vi "19.1-MovingAverage-Window.vi"() -> ()   [LabVIEW 2020]
doc: "This example demonstrates the importance of using windows when performing spectral analysis on signals which contain multiple frequencies.\n\nThe effect of different types of window functions is shown in the frequency domain. With no window function used, Sine Wave 2 buries the low amplitude Sine Wave 1. Using the Hanning Window (Window 2), the smaller signal can be detected."
uses:
  <vilib>/Analysis/0measdsp.llb/Scaled Time Domain Window (DBL).vi
  <vilib>/Analysis/NI_AALPro.lvlib
panel:
  out "H[k]":dbl[][](graph)
  out "H[k]-dB":dbl[][](graph)
  out "h[n]":dbl[][](graph)
  in  "window 1":u32(ring)=5 items=["Rectangle"=0, "Hanning"=1, "Hamming"=2, "Blackman-Harris"=3, "Exact Blackman"=4, "Blackman"=5, "Flat Top"=6, "4 Term B-Harris "=7, "7 Term B-Harris"=8, "Low Sidelobe"=9, "Blackman Nuttall"=11, "Triangle"=30, "Bartlett-Hanning"=31, "Bohman"=32, "Parzen"=33, "Welch"=34, "Kaiser"=60, "Dolph-Chebyshev"=61, "Gaussian"=62]
  in  "window 2":u32(ring)=62 items=["Rectangle"=0, "Hanning"=1, "Hamming"=2, "Blackman-Harris"=3, "Exact Blackman"=4, "Blackman"=5, "Flat Top"=6, "4 Term B-Harris "=7, "7 Term B-Harris"=8, "Low Sidelobe"=9, "Blackman Nuttall"=11, "Triangle"=30, "Bartlett-Hanning"=31, "Bohman"=32, "Parzen"=33, "Welch"=34, "Kaiser"=60, "Dolph-Chebyshev"=61, "Gaussian"=62]
  in  "Stop":bool
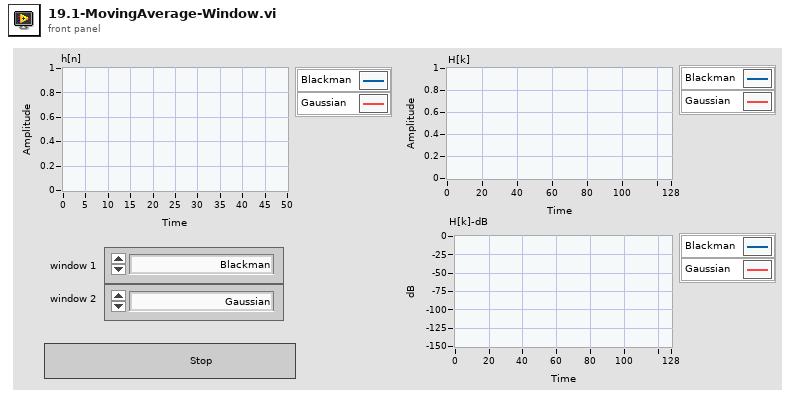
[diagram p1: front panel]
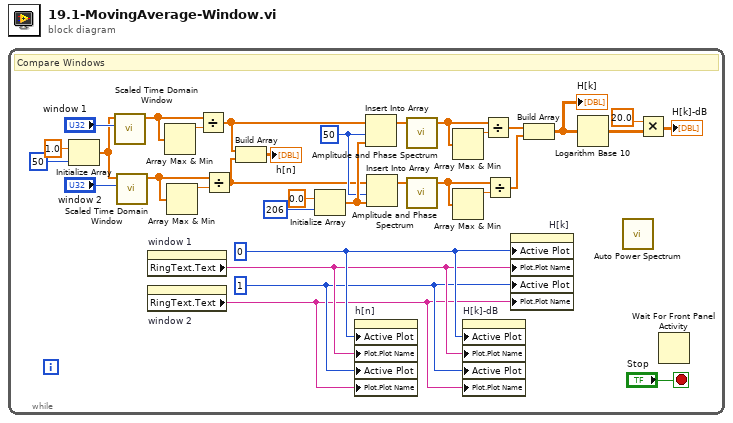
[diagram p0: block diagram]
diagram:
  n1 = while {
    stop <- "Stop" stop-if-true
    w17 = 50 ("index")
    w4 = u32 0
    w2 = u32 1 ("Active Plot")
    # "Compare Windows"
    n2 = Initialize Array(1.0 ("element"), 50 ("dimension size")) -> (w28:dbl[])
    n3 = call-poly <vilib>:"Scaled Time Domain Window.vi"("window"="window 1", "X"=w28) -> ("Windowed X"=w25:dbl[])  [unwired: 7 in, 2 out]
    n4 = call-poly <vilib>:"Scaled Time Domain Window.vi"("window"="window 2", "X"=w28) -> ("Windowed X"=w23:dbl[])  [unwired: 7 in, 2 out]
    n5 = property on="window 1" class="Ring (strict)"() -> ("RingText.Text"=w3:string)  [unwired: 2 in, 2 out]
    n6 = property on="window 2" class="Ring (strict)"() -> ("RingText.Text"=w1:string)  [unwired: 2 in, 2 out]
    n7 = Array Max & Min(array=w25) -> (max value=w26:dbl)  [unwired: 3 out]
    n8 = Array Max & Min(array=w23) -> (max value=w24:dbl)  [unwired: 3 out]
    n9 = Divide(x=w25, y=w26) -> (x/y=w16:dbl[])
    n10 = Divide(x=w23, y=w24) -> (x/y=w15:dbl[])
    n11 = Build Array(w16, w15) -> (→"h[n]":dbl[][])
    n12 = Initialize Array(0.0 ("element"), 206 ("dimension size")) -> (w18:dbl[])
    n13 = property on="h[n]" class="WFGraph (strict)"("Active Plot"=w4, "Plot.Plot Name"=w3, "Active Plot"=w2, "Plot.Plot Name"=w1) -> ()  [unwired: 2 in, 2 out]
    n14 = Insert Into Array(array=w16, index=w17, new element=w18) -> (w12:dbl[])
    n15 = Insert Into Array(array=w15, index=w17, new element=w18) -> (w11:dbl[])
    n16 = call <vilib>:"Amplitude and Phase Spectrum.vi"("Signal (V)"=w12) -> ("Amp Spectrum Mag (Vrms)"=w8:dbl[])  [unwired: 2 in, 2 out]
    n17 = call <vilib>:"Amplitude and Phase Spectrum.vi"("Signal (V)"=w11) -> ("Amp Spectrum Mag (Vrms)"=w7:dbl[])  [unwired: 2 in, 2 out]
    n18 = Array Max & Min(array=w8) -> (max value=w13:dbl)  [unwired: 3 out]
    n19 = Array Max & Min(array=w7) -> (max value=w14:dbl)  [unwired: 3 out]
    n20 = property on="H[k]-dB" class="WFGraph (strict)"("Active Plot"=w4, "Plot.Plot Name"=w3, "Active Plot"=w2, "Plot.Plot Name"=w1) -> ()  [unwired: 2 in, 2 out]
    n21 = Divide(x=w8, y=w13) -> (x/y=w6:dbl[])
    n22 = Divide(x=w7, y=w14) -> (x/y=w5:dbl[])
    n23 = property on="H[k]" class="WFGraph (strict)"("Active Plot"=w4, "Plot.Plot Name"=w3, "Active Plot"=w2, "Plot.Plot Name"=w1) -> ()  [unwired: 2 in, 2 out]
    n24 = Build Array(w6, w5) -> (w9:dbl[][])
    "H[k]" <- w9
    n25 = Logarithm Base 10(1:w9) -> (0:w21:dbl[][])
    n26 = call <vilib>:"Auto Power Spectrum.vi"() -> ()  [unwired: 2 in, 2 out]
    n27 = Multiply(x=20.0, y=w21) -> (x*y=→"H[k]-dB":dbl[][])
    n28 = Wait For Front Panel Activity() -> ()  [unwired: 3 in, 1 out]
  }
